vi "ZedBoardControlsTrippleSwitches.vi"(8 "Str Refnum":refnum<vi>, 9 "Bool Refnum":refnum<vi>, 10 "error out":errorcluster, 11 "queue out":refnum<queue>) -> ()   [LabVIEW 2012]
panel:
  in  "Sync Test\nMode Config":u32
  in  "Pulse Period\n(clock cycles -1)":u32
  in  "Channel \nMux Selector":bool
  in  "Channel \nHold Order":bool
  in  "Channel \nTransfer Order":bool
  in  "Throttle Mode":string(combo)
  in  "Sync Test Mode Select":string(combo)
  in  "Data Input Test Mode":string(combo)
  out "Last Command Sent":string
  out "state 34":bool
  out "state 33":bool
  out "state 32":bool
  in  "Sync2 3B":bool
  in  "Sync1 3B":bool
  in  "Sync0 3B":bool
  out "state 31":bool
  out "state 30":bool
  out "state 29":bool
  in  "Sync2 2B":bool
  in  "Sync1 2B":bool
  in  "Sync0 2B":bool
  out "state 28":bool
  out "state 27":bool
  out "state 26":bool
  in  "Sync2 1B":bool
  in  "Sync1 1B":bool
  in  "Sync0 1B":bool
  out "state 25":bool
  out "state 24":bool
  out "state 23":bool
  in  "Sync2 0B":bool
  in  "Sync1 0B":bool
  in  "Sync0 0B":bool
  out "state 22":bool
  out "state 21":bool
  out "state 20":bool
  in  "Sync2 7":bool
  in  "Sync1 7":bool
  in  "Sync0 7":bool
  out "state 19":bool
  out "state 18":bool
  out "state 17":bool
  in  "Sync2 6":bool
  in  "Sync1 6":bool
  in  "Sync0 6":bool
  out "state 16":bool
  out "state 15":bool
  out "state 14":bool
  in  "Sync2 5":bool
  in  "Sync1 5":bool
  in  "Sync0 5":bool
  out "state 13":bool
  out "state 12":bool
  out "state 11":bool
  in  "Sync2 4":bool
  in  "Sync1 4":bool
  in  "Sync0 4":bool
  out "state 10":bool
  out "state 9":bool
  out "state 8":bool
  in  "Sync2 3A":bool
  in  "Sync13A":bool
  in  "Sync0 3A":bool
  out "state 7":bool
  out "state 6":bool
  out "state 5":bool
  in  "Sync2 2A":bool
  in  "Sync1 2A":bool
  in  "Sync0 2A":bool
  out "state 4":bool
  out "state 2":bool
  out "state 3":bool
  in  "Sync2 1A":bool
  in  "Sync1 1A":bool
  in  "Sync0 1A":bool
  out "state":bool
  out "state 35":bool
  out "state 36":bool
  in  "Sync2 0A":bool
  in  "Sync1 0A":bool
  in  "Sync0 0A":bool
  in  "Reset Channel Enable":bool
  in  "Send Command, manual entry":string
  in  "Send":bool
  in  "Read Register":bool
  in  "Reset Register Map to Defaults":bool
  in  "Sync Enable":bool[](array[boolean])
  in  "Channel Enable":bool[](array[boolean])
  in  "Reset Profile Accumulator":bool[](array[boolean])
  in  "Counts Per Bin":u16
  in  "User Reset":bool
  in  "Number of Bins":u16
  in  "Profiles Per Histogram":u16
  in  "Time Reset":bool
  in  "Relative Time Step":u32
  in  "Demux Channel Enable":bool[](array[boolean])
  out "word0":string
  out "word1":string
  out "word2":string
  out "word3":string
  out "word4":string
  out "word5":string
  out "word6":string
  out "word7":string
  out "word8":string
  in  "Channel Polarization":bool[](array[boolean])
  in  "Demux Polarization":bool[](array[boolean])
  in  "Sync Polarization":bool[](array[boolean])
  in  "PIN0 Pulse Durration Ave 2^N":u16
  out "word9":string
  in  "PIN1 Pulse Durration Ave 2^N":u16
  in  "PIN2 Pulse Durration Ave 2^N":u16
  in  "PIN3 Pulse Durration Ave 2^N":u16
  in  "PIN4 Pulse Durration Ave 2^N":u16
  in  "PIN5 Pulse Durration Ave 2^N":u16
  in  "Send Word 0":bool
  in  "Send Word 1":bool
  in  "Send Word 2":bool
  in  "Send Word 3":bool
  in  "Send Word 4":bool
  in  "Send Word 5":bool
  in  "Send Word 6":bool
  in  "Send Word 7":bool
  in  "Send Word 8":bool
  in  "Send Word 9":bool
  # "word0"
  # "word1"
  # "word2"
  # "word3"
  # "word4"
  # "valid range (2-4096)"
  # "valid range (2-4096)"
  # "valid range (1-32,768)"
  # "word6"
  # "valid range (0-256)"
  # "valid range (0-128)"
  # "word7"
  # "word8"
  # "valid range (0-33,554,432)"
  # "word9"
  # "N=valid range (0-15)"
  # "N=valid range (0-15)"
  # "N=valid range (0-15)"
  # "N=valid range (0-15)"
  # "N=valid range (0-15)"
  # "N=valid range (0-15)"
  # "word5"
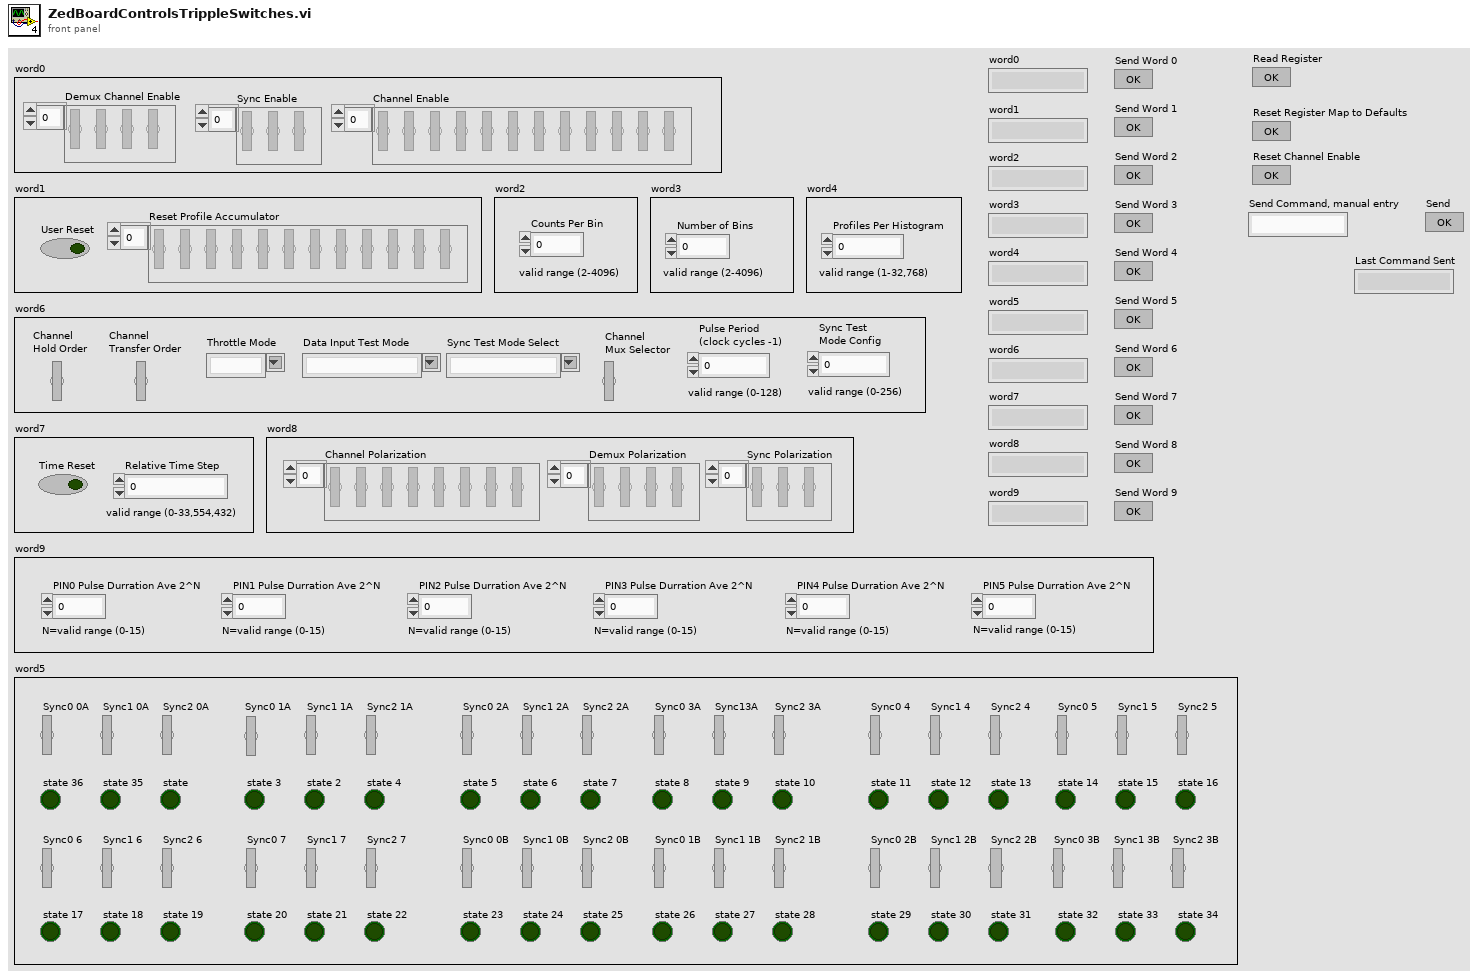
[diagram p1: front panel]
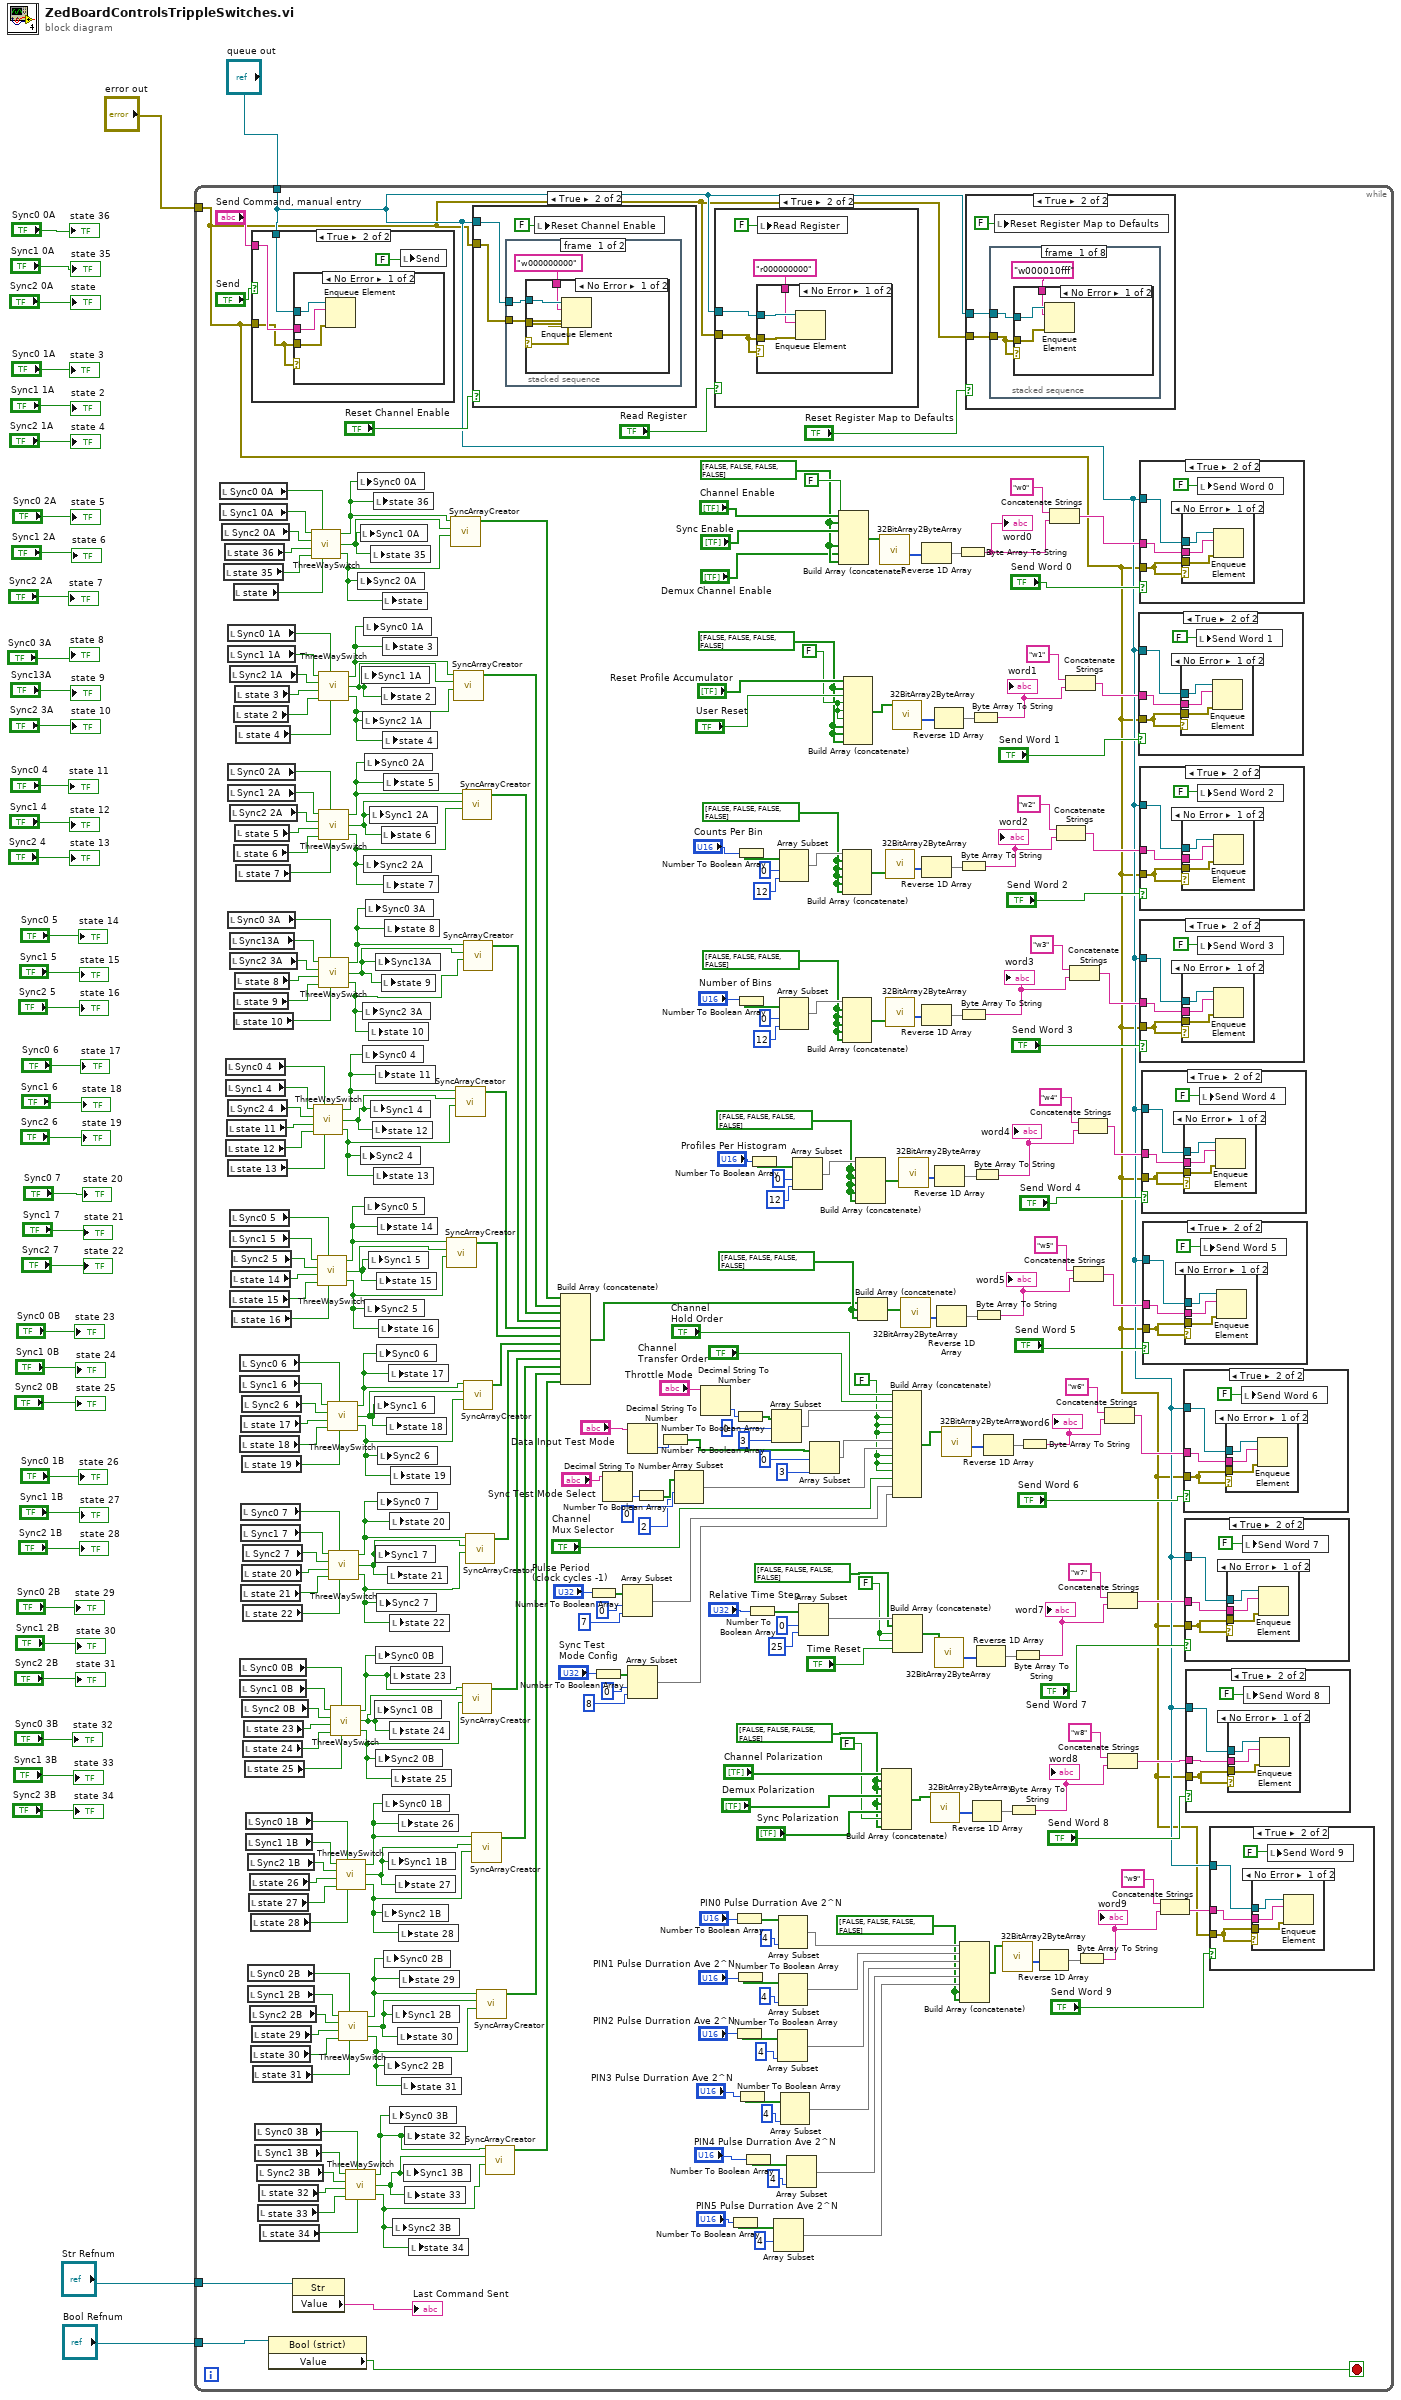
[diagram p0: block diagram]
diagram:
  n1 = while {
    tunnel: "queue out" -> [w200]
    tunnel: "error out" -> [w198]
    tunnel: "Bool Refnum" -> [w75]
    tunnel: "Str Refnum" -> [w73]
    stop <- w74 stop-if-true
    w239 = bool[] [FALSE, FALSE, FALSE, FALSE] ("appended array")
    w266 = bool[] [FALSE, FALSE, FALSE, FALSE] ("appended array")
    w275 = FALSE ("Read Register")
    w48 = FALSE ("Read Register")
    w287 = bool[] [FALSE, FALSE, FALSE, FALSE] ("appended array")
    w283 = bool[] [FALSE, FALSE, FALSE, FALSE] ("appended array")
    w284 = bool[] [FALSE, FALSE, FALSE, FALSE] ("appended array")
    w285 = bool[] [FALSE, FALSE, FALSE, FALSE] ("appended array")
    w311 = FALSE ("Read Register")
    w310 = bool[] [FALSE, FALSE, FALSE, FALSE] ("appended array")
    w320 = bool[] [FALSE, FALSE, FALSE, FALSE] ("appended array")
    n2 = local read "Sync0 0A"() -> (w170:bool)
    n3 = local read "Sync1 0A"() -> (w171:bool)
    n4 = local read "Sync2 0A"() -> (w172:bool)
    n5 = local read "state 35"() -> (w168:bool)
    n6 = local read "state 36"() -> (w167:bool)
    n7 = local read "Sync0 4"() -> (w175:bool)
    n8 = local read "Sync1 4"() -> (w174:bool)
    n9 = local read "state 12"() -> (w177:bool)
    n10 = local read "state 11"() -> (w178:bool)
    n11 = local read "Sync0 1A"() -> (w194:bool)
    n12 = local read "Sync1 1A"() -> (w195:bool)
    n13 = local read "Sync0 2A"() -> (w187:bool)
    n14 = local read "Sync1 2A"() -> (w186:bool)
    n15 = local read "Sync0 3A"() -> (w181:bool)
    n16 = local read "Sync2 4"() -> (w173:bool)
    n17 = local read "state 13"() -> (w176:bool)
    n18 = local read "Sync2 1A"() -> (w196:bool)
    n19 = local read "Sync2 2A"() -> (w185:bool)
    n20 = local read "Sync13A"() -> (w180:bool)
    n21 = local read "Sync2 3A"() -> (w179:bool)
    n22 = local read "Sync0 5"() -> (w164:bool)
    n23 = local read "Sync1 5"() -> (w165:bool)
    n24 = local read "state 15"() -> (w162:bool)
    n25 = local read "state 14"() -> (w161:bool)
    n26 = local read "Sync2 5"() -> (w166:bool)
    n27 = local read "state 16"() -> (w163:bool)
    n28 = local read "state"() -> (w169:bool)
    n29 = local read "state 10"() -> (w182:bool)
    n30 = local read "state 2"() -> (w192:bool)
    n31 = local read "state 6"() -> (w189:bool)
    n32 = local read "state 9"() -> (w183:bool)
    n33 = local read "state 3"() -> (w191:bool)
    n34 = local read "state 5"() -> (w190:bool)
    n35 = local read "state 8"() -> (w184:bool)
    n36 = local read "state 4"() -> (w193:bool)
    n37 = local read "state 7"() -> (w188:bool)
    n38 = local read "Sync0 6"() -> (w157:bool)
    n39 = local read "Sync1 6"() -> (w156:bool)
    n40 = local read "state 18"() -> (w159:bool)
    n41 = local read "Sync0 0B"() -> (w145:bool)
    n42 = local read "Sync1 0B"() -> (w144:bool)
    n43 = local read "state 17"() -> (w160:bool)
    n44 = local read "Sync0 7"() -> (w152:bool)
    n45 = local read "Sync1 7"() -> (w153:bool)
    n46 = local read "state 21"() -> (w150:bool)
    n47 = local read "Sync2 6"() -> (w155:bool)
    n48 = local read "state 19"() -> (w158:bool)
    n49 = local read "state 20"() -> (w149:bool)
    n50 = local read "Sync2 0B"() -> (w143:bool)
    n51 = local read "Sync2 7"() -> (w154:bool)
    n52 = local read "state 22"() -> (w151:bool)
    n53 = local read "state 24"() -> (w147:bool)
    n54 = local read "state 23"() -> (w148:bool)
    n55 = local read "state 25"() -> (w146:bool)
    n56 = local read "Sync0 1B"() -> (w140:bool)
    n57 = local read "Sync1 1B"() -> (w141:bool)
    n58 = local read "Sync2 1B"() -> (w142:bool)
    n59 = local read "Sync0 2B"() -> (w133:bool)
    n60 = local read "Sync1 2B"() -> (w132:bool)
    n61 = local read "state 27"() -> (w138:bool)
    n62 = local read "state 26"() -> (w137:bool)
    n63 = local read "Sync2 2B"() -> (w131:bool)
    n64 = local read "state 28"() -> (w139:bool)
    n65 = local read "state 30"() -> (w135:bool)
    n66 = case shown="True" "Send" {
      tunnel: "Send Command, manual entry" -> [_ w487]
      tunnel: w200 -> [_ w486]
      tunnel: w198 -> [_ w484]
      frame False {
      }
      frame True {
        n67 = case shown="No Error" w484 {
          tunnel: w487 -> [w490 _]
          tunnel: w484 -> [w489 _]
          tunnel: w486 -> [w488 _]
          frame No Error {
            n68 = Enqueue Element(queue=w488, element=w490, error in (no error)=w489) -> ()  [unwired: 1 in, 3 out]
          }
          frame Error {
          }
        }
        n69 = local write "Send"(FALSE ("Send")) -> ()
      }
    }
    n70 = local read "state 29"() -> (w136:bool)
    n71 = local read "state 31"() -> (w134:bool)
    n72 = local read "Sync0 3B"() -> (w128:bool)
    n73 = local read "Sync1 3B"() -> (w129:bool)
    n74 = local read "Sync2 3B"() -> (w130:bool)
    n75 = local read "state 33"() -> (w126:bool)
    n76 = local read "state 32"() -> (w125:bool)
    n77 = local read "state 34"() -> (w127:bool)
    n78 = property class="Bool (strict)"(reference=w75) -> ("Value"=w74:bool)  [unwired: 1 in, 2 out]
    n79 = property class="Str"(reference=w73) -> ("Value"=→"Last Command Sent":string)  [unwired: 1 in, 2 out]
    n80 = call "ThreeWaySwitch.vi"("Sync1"=w171, "Sync0"=w170, "Sync2"=w172, "Sync0 last state"=w167, "Sync2 last state"=w169, "Sync1 last state"=w168) -> ("Sync0out"=w124:bool, "Sync1out"=w123:bool, "Sync2out"=w122:bool)
    n81 = call "ThreeWaySwitch.vi"("Sync1"=w174, "Sync0"=w175, "Sync2"=w173, "Sync0 last state"=w178, "Sync2 last state"=w176, "Sync1 last state"=w177) -> ("Sync0out"=w112:bool, "Sync1out"=w111:bool, "Sync2out"=w110:bool)
    n82 = call "ThreeWaySwitch.vi"("Sync1"=w165, "Sync0"=w164, "Sync2"=w166, "Sync0 last state"=w161, "Sync2 last state"=w163, "Sync1 last state"=w162) -> ("Sync0out"=w109:bool, "Sync1out"=w108:bool, "Sync2out"=w107:bool)
    n83 = call "ThreeWaySwitch.vi"("Sync1"=w195, "Sync0"=w194, "Sync2"=w196, "Sync0 last state"=w191, "Sync2 last state"=w193, "Sync1 last state"=w192) -> ("Sync0out"=w119:bool, "Sync1out"=w120:bool, "Sync2out"=w121:bool)
    n84 = call "ThreeWaySwitch.vi"("Sync1"=w186, "Sync0"=w187, "Sync2"=w185, "Sync0 last state"=w190, "Sync2 last state"=w188, "Sync1 last state"=w189) -> ("Sync0out"=w118:bool, "Sync1out"=w117:bool, "Sync2out"=w116:bool)
    n85 = call "ThreeWaySwitch.vi"("Sync1"=w180, "Sync0"=w181, "Sync2"=w179, "Sync0 last state"=w184, "Sync2 last state"=w182, "Sync1 last state"=w183) -> ("Sync0out"=w115:bool, "Sync1out"=w114:bool, "Sync2out"=w113:bool)
    n86 = call "ThreeWaySwitch.vi"("Sync1"=w156, "Sync0"=w157, "Sync2"=w155, "Sync0 last state"=w160, "Sync2 last state"=w158, "Sync1 last state"=w159) -> ("Sync0out"=w106:bool, "Sync1out"=w105:bool, "Sync2out"=w104:bool)
    n87 = call "ThreeWaySwitch.vi"("Sync1"=w153, "Sync0"=w152, "Sync2"=w154, "Sync0 last state"=w149, "Sync2 last state"=w151, "Sync1 last state"=w150) -> ("Sync0out"=w103:bool, "Sync1out"=w102:bool, "Sync2out"=w101:bool)
    n88 = call "ThreeWaySwitch.vi"("Sync1"=w144, "Sync0"=w145, "Sync2"=w143, "Sync0 last state"=w148, "Sync2 last state"=w146, "Sync1 last state"=w147) -> ("Sync0out"=w100:bool, "Sync1out"=w99:bool, "Sync2out"=w98:bool)
    n89 = call "ThreeWaySwitch.vi"("Sync1"=w141, "Sync0"=w140, "Sync2"=w142, "Sync0 last state"=w137, "Sync2 last state"=w139, "Sync1 last state"=w138) -> ("Sync0out"=w97:bool, "Sync1out"=w96:bool, "Sync2out"=w95:bool)
    n90 = call "ThreeWaySwitch.vi"("Sync1"=w132, "Sync0"=w133, "Sync2"=w131, "Sync0 last state"=w136, "Sync2 last state"=w134, "Sync1 last state"=w135) -> ("Sync0out"=w94:bool, "Sync1out"=w93:bool, "Sync2out"=w92:bool)
    n91 = call "ThreeWaySwitch.vi"("Sync1"=w129, "Sync0"=w128, "Sync2"=w130, "Sync0 last state"=w125, "Sync2 last state"=w127, "Sync1 last state"=w126) -> ("Sync0out"=w91:bool, "Sync1out"=w90:bool, "Sync2out"=w89:bool)
    n92 = local write "Sync0 0A"(w124) -> ()
    n93 = local write "Sync2 0A"(w122) -> ()
    n94 = local write "Sync1 0A"(w123) -> ()
    n95 = local write "Sync2 4"(w110) -> ()
    n96 = local write "Sync1 1A"(w120) -> ()
    n97 = local write "Sync2 1A"(w121) -> ()
    n98 = local write "Sync2 3A"(w113) -> ()
    n99 = local write "Sync0 4"(w112) -> ()
    n100 = local write "Sync0 1A"(w119) -> ()
    n101 = local write "Sync2 2A"(w116) -> ()
    n102 = local write "Sync0 2A"(w118) -> ()
    n103 = local write "Sync0 5"(w109) -> ()
    n104 = local write "Sync2 5"(w107) -> ()
    n105 = local write "Sync0 3A"(w115) -> ()
    n106 = local write "state 10"(w113) -> ()
    n107 = local write "Sync1 5"(w108) -> ()
    n108 = local write "Sync1 2A"(w117) -> ()
    n109 = local write "state 35"(w123) -> ()
    n110 = local write "Sync1 4"(w111) -> ()
    n111 = local write "state 12"(w111) -> ()
    n112 = local write "state 36"(w124) -> ()
    n113 = local write "state 13"(w110) -> ()
    n114 = local write "Sync1 6"(w105) -> ()
    n115 = local write "Sync1 0B"(w99) -> ()
    n116 = local write "Sync13A"(w114) -> ()
    n117 = local write "state 11"(w112) -> ()
    n118 = local write "Sync1 7"(w102) -> ()
    n119 = local write "Sync0 0B"(w100) -> ()
    n120 = local write "Sync2 0B"(w98) -> ()
    n121 = local write "state 15"(w108) -> ()
    n122 = local write "Sync0 6"(w106) -> ()
    n123 = local write "Sync2 7"(w101) -> ()
    n124 = local write "state 14"(w109) -> ()
    n125 = local write "Sync2 6"(w104) -> ()
    n126 = local write "Sync0 7"(w103) -> ()
    n127 = local write "state 16"(w107) -> ()
    n128 = local write "state 2"(w120) -> ()
    n129 = local write "state 6"(w117) -> ()
    n130 = local write "state 9"(w114) -> ()
    n131 = local write "state"(w122) -> ()
    n132 = local write "Sync2 1B"(w95) -> ()
    n133 = local write "state 3"(w119) -> ()
    n134 = local write "state 4"(w121) -> ()
    n135 = local write "Sync0 1B"(w97) -> ()
    n136 = local write "state 5"(w118) -> ()
    n137 = local write "state 7"(w116) -> ()
    n138 = local write "Sync0 2B"(w94) -> ()
    n139 = local write "state 8"(w115) -> ()
    n140 = local write "Sync2 2B"(w92) -> ()
    n141 = local write "state 18"(w105) -> ()
    n142 = local write "state 21"(w102) -> ()
    n143 = local write "state 17"(w106) -> ()
    n144 = local write "Sync1 1B"(w96) -> ()
    n145 = local write "state 20"(w103) -> ()
    n146 = local write "state 22"(w101) -> ()
    n147 = local write "state 24"(w99) -> ()
    n148 = local write "Sync0 3B"(w91) -> ()
    n149 = local write "state 19"(w104) -> ()
    n150 = local write "state 23"(w100) -> ()
    n151 = local write "state 25"(w98) -> ()
    n152 = local write "Sync1 2B"(w93) -> ()
    n153 = local write "Sync2 3B"(w89) -> ()
    n154 = local write "state 27"(w96) -> ()
    n155 = local write "state 30"(w93) -> ()
    n156 = local write "state 26"(w97) -> ()
    n157 = local write "state 28"(w95) -> ()
    n158 = local write "state 29"(w94) -> ()
    n159 = local write "state 31"(w92) -> ()
    n160 = local write "Sync1 3B"(w90) -> ()
    n161 = local write "state 32"(w91) -> ()
    n162 = local write "state 33"(w90) -> ()
    n163 = local write "state 34"(w89) -> ()
    n164 = call "SyncArrayCreator.vi"("Sync2"=w107, "Sync1"=w108, "Sync0"=w109) -> ("Array"=w83:bool[])  [unwired: 8 in]
    n165 = call "SyncArrayCreator.vi"("Sync2"=w122, "Sync1"=w123, "Sync0"=w124) -> ("Array"=w88:bool[])  [unwired: 8 in]
    n166 = call "SyncArrayCreator.vi"("Sync2"=w121, "Sync1"=w120, "Sync0"=w119) -> ("Array"=w87:bool[])  [unwired: 8 in]
    n167 = call "SyncArrayCreator.vi"("Sync2"=w110, "Sync1"=w111, "Sync0"=w112) -> ("Array"=w84:bool[])  [unwired: 8 in]
    n168 = call "SyncArrayCreator.vi"("Sync2"=w116, "Sync1"=w117, "Sync0"=w118) -> ("Array"=w86:bool[])  [unwired: 8 in]
    n169 = call "SyncArrayCreator.vi"("Sync2"=w98, "Sync1"=w99, "Sync0"=w100) -> ("Array"=w80:bool[])  [unwired: 8 in]
    n170 = call "SyncArrayCreator.vi"("Sync2"=w113, "Sync1"=w114, "Sync0"=w115) -> ("Array"=w85:bool[])  [unwired: 8 in]
    n171 = call "SyncArrayCreator.vi"("Sync2"=w104, "Sync1"=w105, "Sync0"=w106) -> ("Array"=w82:bool[])  [unwired: 8 in]
    n172 = call "SyncArrayCreator.vi"("Sync2"=w101, "Sync1"=w102, "Sync0"=w103) -> ("Array"=w81:bool[])  [unwired: 8 in]
    n173 = call "SyncArrayCreator.vi"("Sync2"=w95, "Sync1"=w96, "Sync0"=w97) -> ("Array"=w79:bool[])  [unwired: 8 in]
    n174 = case shown="True" "Reset Channel Enable" {
      tunnel: w198 -> [_ w469]
      tunnel: w200 -> [_ w470]
      frame False {
      }
      frame True {
        n175 = stacked-sequence {
          tunnel: w469 -> [w474 w479]
          tunnel: w470 -> [w472 w478]
          frame #0 {
            n176 = case shown="No Error" w474 {
              tunnel: w474 -> [w477 _]
              tunnel: w472 -> [w476 _]
              tunnel: "w000000000" ("F-format string") -> [w475 _]
              frame No Error {
                n177 = Enqueue Element(queue=w476, element=w475, error in (no error)=w477) -> ()  [unwired: 1 in, 3 out]
              }
              frame Error {
              }
            }
          }
          frame #1 {
            n178 = case shown="No Error" w479 {
              tunnel: "w000010fff" ("F-format string") -> [w483 _]
              tunnel: w478 -> [w482 _]
              tunnel: w479 -> [w481 _]
              frame No Error {
                n179 = Enqueue Element(queue=w482, element=w483, error in (no error)=w481) -> ()  [unwired: 1 in, 3 out]
              }
              frame Error {
              }
            }
          }
        }
        n180 = local write "Reset Channel Enable"(FALSE ("Reset")) -> ()
      }
    }
    n181 = call "SyncArrayCreator.vi"("Sync2"=w92, "Sync1"=w93, "Sync0"=w94) -> ("Array"=w78:bool[])  [unwired: 8 in]
    n182 = call "SyncArrayCreator.vi"("Sync2"=w89, "Sync1"=w90, "Sync0"=w91) -> ("Array"=w77:bool[])  [unwired: 8 in]
    n183 = Build Array (concatenate)(w88, w87, w86, w85, w84, w83, w82, w81, w80, w79, w78, w77) -> (w76:bool[])
    n184 = Number To Boolean Array(number="Pulse Period\n(clock cycles -1)") -> (Boolean array=w59:bool[])
    n185 = Number To Boolean Array(number="Sync Test\nMode Config") -> (Boolean array=w46:bool[])
    n186 = Decimal String To Number(string="Sync Test Mode Select") -> (number=w66:i32)  [unwired: 2 in, 1 out]
    n187 = Array Subset(array=w59, index=0, length=7) -> (w51:bool[])
    n188 = Decimal String To Number(string="Data Input Test Mode") -> (number=w67:i32)  [unwired: 2 in, 1 out]
    n189 = Array Subset(array=w46, index=0, length=8) -> (w42:bool[])
    n190 = Number To Boolean Array(number=w66) -> (Boolean array=w60:bool[])
    n191 = Number To Boolean Array(number=w67) -> (Boolean array=w61:bool[])
    n192 = Array Subset(array=w60, index=0, length=2) -> (w49:bool[])
    n193 = Decimal String To Number(string="Throttle Mode") -> (number=w70:i32)  [unwired: 2 in, 1 out]
    n194 = case shown="True" "Read Register" {
      tunnel: w200 -> [_ w464]
      tunnel: w198 -> [_ w463]
      frame False {
      }
      frame True {
        n195 = case shown="No Error" w463 {
          tunnel: w464 -> [w468 _]
          tunnel: w463 -> [w467 _]
          tunnel: "r000000000" ("F-format string") -> [w466 _]
          frame No Error {
            n196 = Enqueue Element(queue=w468, element=w466, error in (no error)=w467) -> ()  [unwired: 1 in, 3 out]
          }
          frame Error {
          }
        }
        n197 = local write "Read Register"(FALSE ("Read Register")) -> ()
      }
    }
    n198 = Number To Boolean Array(number="PIN5 Pulse Durration Ave 2^N") -> (Boolean array=w255:bool[])
    n199 = Number To Boolean Array(number="PIN0 Pulse Durration Ave 2^N") -> (Boolean array=w264:bool[])
    n200 = Number To Boolean Array(number="PIN2 Pulse Durration Ave 2^N") -> (Boolean array=w251:bool[])
    n201 = Number To Boolean Array(number=w70) -> (Boolean array=w330:bool[])
    n202 = Number To Boolean Array(number="PIN1 Pulse Durration Ave 2^N") -> (Boolean array=w259:bool[])
    n203 = Number To Boolean Array(number="Counts Per Bin") -> (Boolean array=w333:bool[])
    n204 = Number To Boolean Array(number="Number of Bins") -> (Boolean array=w304:bool[])
    n205 = Number To Boolean Array(number="PIN3 Pulse Durration Ave 2^N") -> (Boolean array=w253:bool[])
    n206 = Number To Boolean Array(number="PIN4 Pulse Durration Ave 2^N") -> (Boolean array=w257:bool[])
    n207 = Number To Boolean Array(number="Relative Time Step") -> (Boolean array=w327:bool[])
    n208 = Number To Boolean Array(number="Profiles Per Histogram") -> (Boolean array=w296:bool[])
    n209 = Array Subset(array=w330, index=0, length=3) -> (w55:bool[])
    n210 = Array Subset(array=w255, length=4) -> (w240:bool[])  [unwired: 1 in]
    n211 = Array Subset(array=w251, length=4) -> (w243:bool[])  [unwired: 1 in]
    n212 = Array Subset(array=w264, length=4) -> (w245:bool[])  [unwired: 1 in]
    n213 = Array Subset(array=w259, length=4) -> (w244:bool[])  [unwired: 1 in]
    n214 = Array Subset(array=w333, index=0, length=12) -> (w307:bool[])
    n215 = Array Subset(array=w304, index=0, length=12) -> (w300:bool[])
    n216 = Array Subset(array=w253, length=4) -> (w242:bool[])  [unwired: 1 in]
    n217 = Array Subset(array=w257, length=4) -> (w241:bool[])  [unwired: 1 in]
    n218 = Array Subset(array=w296, index=0, length=12) -> (w292:bool[])
    n219 = Array Subset(array=w327, index=0, length=25) -> (w277:bool[])
    n220 = Array Subset(array=w61, index=0, length=3) -> (w52:bool[])
    n221 = Build Array (concatenate)("Channel Enable", w320, "Sync Enable", FALSE ("Read Register"), w320, "Demux Channel Enable", w320) -> (w324:bool[])
    n222 = Build Array (concatenate)(w307, w285, w285, w285, w285, w285) -> (w286:bool[])
    n223 = Build Array (concatenate)(w300, w284, w284, w284, w284, w284) -> (w303:bool[])
    n224 = Build Array (concatenate)("Reset Profile Accumulator", w310, "User Reset", w311, w311, w311, w310, w310, w310) -> (w316:bool[])
    n225 = Build Array (concatenate)(w292, w283, w283, w283, w283, w283) -> (w295:bool[])
    n226 = Build Array (concatenate)(w76, w287, w287) -> (w290:bool[])
    n227 = call "32BitArray2ByteArray.vi"("Array in"=w324) -> ("Byte array out"=w318:u32[])  [unwired: 10 in]
    n228 = Build Array (concatenate)("Channel Polarization", w266, w266, "Demux Polarization", w266, "Sync Polarization", FALSE ("Read Register"), w266) -> (w273:bool[])
    n229 = call "32BitArray2ByteArray.vi"("Array in"=w286) -> ("Byte array out"=w309:u32[])  [unwired: 10 in]
    n230 = call "32BitArray2ByteArray.vi"("Array in"=w303) -> ("Byte array out"=w302:u32[])  [unwired: 10 in]
    n231 = call "32BitArray2ByteArray.vi"("Array in"=w316) -> ("Byte array out"=w315:u32[])  [unwired: 10 in]
    n232 = Build Array (concatenate)("Channel \nHold Order", "Channel \nTransfer Order", w55, w48, w48, w48, w52, w49, w48, w48, w48, "Channel \nMux Selector", w51, w42) -> (w47:bool[])
    n233 = Build Array (concatenate)(w277, bool[] [FALSE, FALSE, FALSE, FALSE] ("appended array"), w275, w275, "Time Reset") -> (w280:bool[])
    n234 = call "32BitArray2ByteArray.vi"("Array in"=w295) -> ("Byte array out"=w294:u32[])  [unwired: 10 in]
    n235 = call "32BitArray2ByteArray.vi"("Array in"=w290) -> ("Byte array out"=w289:u32[])  [unwired: 10 in]
    n236 = Reverse 1D Array(array=w318) -> (reversed array=w317:u32[])
    n237 = Reverse 1D Array(array=w309) -> (reversed array=w308:u32[])
    n238 = Reverse 1D Array(array=w302) -> (reversed array=w301:u32[])
    n239 = call "32BitArray2ByteArray.vi"("Array in"=w273) -> ("Byte array out"=w272:u32[])  [unwired: 10 in]
    n240 = Reverse 1D Array(array=w315) -> (reversed array=w314:u32[])
    n241 = call "32BitArray2ByteArray.vi"("Array in"=w280) -> ("Byte array out"=w279:u32[])  [unwired: 10 in]
    n242 = Reverse 1D Array(array=w294) -> (reversed array=w293:u32[])
    n243 = Reverse 1D Array(array=w289) -> (reversed array=w288:u32[])
    n244 = call "32BitArray2ByteArray.vi"("Array in"=w47) -> ("Byte array out"=w282:u32[])  [unwired: 10 in]
    n245 = Byte Array To String(unsigned byte array=w317) -> (string=w237:string)
    "word0" <- w237
    n246 = Byte Array To String(unsigned byte array=w308) -> (string=w222:string)
    "word2" <- w222
    n247 = Byte Array To String(unsigned byte array=w301) -> (string=w215:string)
    "word3" <- w215
    n248 = Build Array (concatenate)(w245, w244, w243, w242, w241, w240, w239, w239) -> (w263:bool[])
    n249 = case shown="True" "Reset Register Map to Defaults" {
      tunnel: w200 -> [_ w412]
      tunnel: w198 -> [_ w411]
      frame False {
      }
      frame True {
        n250 = stacked-sequence {
          tunnel: w412 -> [w416 w422 w428 w434 w440 w446 w452 w458]
          tunnel: w411 -> [w415 w421 w427 w433 w439 w445 w451 w457]
          frame #0 {
            n251 = case shown="No Error" w415 {
              tunnel: w416 -> [w419 _]
              tunnel: w415 -> [w418 _]
              tunnel: "w000010fff" ("F-format string") -> [w417 _]
              frame No Error {
                n252 = Enqueue Element(queue=w419, element=w417, error in (no error)=w418) -> ()  [unwired: 1 in, 3 out]
              }
              frame Error {
              }
            }
          }
          frame #1 {
            n253 = case shown="No Error" w421 {
              tunnel: w422 -> [w425 _]
              tunnel: w421 -> [w424 _]
              tunnel: "w100000000" ("F-format string") -> [w423 _]
              frame No Error {
                n254 = Enqueue Element(queue=w425, element=w423, error in (no error)=w424) -> ()  [unwired: 1 in, 3 out]
              }
              frame Error {
              }
            }
          }
          frame #2 {
            n255 = case shown="No Error" w427 {
              tunnel: w428 -> [w431 _]
              tunnel: w427 -> [w430 _]
              tunnel: "w20000000a" ("F-format string") -> [w429 _]
              frame No Error {
                n256 = Enqueue Element(queue=w431, element=w429, error in (no error)=w430) -> ()  [unwired: 1 in, 3 out]
              }
              frame Error {
              }
            }
          }
          frame #3 {
            n257 = case shown="No Error" w433 {
              tunnel: w434 -> [w437 _]
              tunnel: w433 -> [w436 _]
              tunnel: "w300000bb8" ("F-format string") -> [w435 _]
              frame No Error {
                n258 = Enqueue Element(queue=w437, element=w435, error in (no error)=w436) -> ()  [unwired: 1 in, 3 out]
              }
              frame Error {
              }
            }
          }
          frame #4 {
            n259 = case shown="No Error" w439 {
              tunnel: w440 -> [w443 _]
              tunnel: w439 -> [w442 _]
              tunnel: "w400002000" ("F-format string") -> [w441 _]
              frame No Error {
                n260 = Enqueue Element(queue=w443, element=w441, error in (no error)=w442) -> ()  [unwired: 1 in, 3 out]
              }
              frame Error {
              }
            }
          }
          frame #5 {
            n261 = case shown="No Error" w445 {
              tunnel: w446 -> [w449 _]
              tunnel: w445 -> [w448 _]
              tunnel: "w500000000" ("F-format string") -> [w447 _]
              frame No Error {
                n262 = Enqueue Element(queue=w449, element=w447, error in (no error)=w448) -> ()  [unwired: 1 in, 3 out]
              }
              frame Error {
              }
            }
          }
          frame #6 {
            n263 = case shown="No Error" w451 {
              tunnel: w452 -> [w455 _]
              tunnel: w451 -> [w454 _]
              tunnel: "w61f000a00" ("F-format string") -> [w453 _]
              frame No Error {
                n264 = Enqueue Element(queue=w455, element=w453, error in (no error)=w454) -> ()  [unwired: 1 in, 3 out]
              }
              frame Error {
              }
            }
          }
          frame #7 {
            n265 = case shown="No Error" w457 {
              tunnel: w458 -> [w461 _]
              tunnel: w457 -> [w460 _]
              tunnel: "w701312d00" ("F-format string") -> [w459 _]
              frame No Error {
                n266 = Enqueue Element(queue=w461, element=w459, error in (no error)=w460) -> ()  [unwired: 1 in, 3 out]
              }
              frame Error {
              }
            }
          }
        }
        n267 = local write "Reset Register Map to Defaults"(FALSE ("Read Register")) -> ()
      }
    }
    n268 = Byte Array To String(unsigned byte array=w314) -> (string=w225:string)
    "word1" <- w225
    n269 = Byte Array To String(unsigned byte array=w293) -> (string=w216:string)
    "word4" <- w216
    n270 = Reverse 1D Array(array=w272) -> (reversed array=w271:u32[])
    n271 = Byte Array To String(unsigned byte array=w288) -> (string=w217:string)
    "word5" <- w217
    n272 = Reverse 1D Array(array=w279) -> (reversed array=w278:u32[])
    n273 = Reverse 1D Array(array=w282) -> (reversed array=w281:u32[])
    n274 = call "32BitArray2ByteArray.vi"("Array in"=w263) -> ("Byte array out"=w262:u32[])  [unwired: 10 in]
    n275 = Byte Array To String(unsigned byte array=w271) -> (string=w220:string)
    "word8" <- w220
    n276 = Byte Array To String(unsigned byte array=w278) -> (string=w219:string)
    "word7" <- w219
    n277 = Byte Array To String(unsigned byte array=w281) -> (string=w218:string)
    "word6" <- w218
    n278 = Reverse 1D Array(array=w262) -> (reversed array=w261:u32[])
    n279 = Concatenate Strings("w0" ("string"), w237) -> (w236:string)
    n280 = Concatenate Strings("w2" ("string"), w222) -> (w214:string)
    n281 = Concatenate Strings("w1" ("string"), w225) -> (w223:string)
    n282 = Concatenate Strings("w3" ("string"), w215) -> (w213:string)
    n283 = Concatenate Strings("w5" ("string"), w217) -> (w211:string)
    n284 = Byte Array To String(unsigned byte array=w261) -> (string=w221:string)
    "word9" <- w221
    n285 = Concatenate Strings("w4" ("string"), w216) -> (w212:string)
    n286 = Concatenate Strings("w6" ("string"), w218) -> (w210:string)
    n287 = Concatenate Strings("w7" ("string"), w219) -> (w203:string)
    n288 = Concatenate Strings("w8" ("string"), w220) -> (w201:string)
    n289 = case shown="True" "Send Word 1" {
      tunnel: w223 -> [_ w400]
      tunnel: w200 -> [_ w399]
      tunnel: w198 -> [_ w397]
      frame False {
      }
      frame True {
        n290 = case shown="No Error" w397 {
          tunnel: w400 -> [w403 _]
          tunnel: w397 -> [w402 _]
          tunnel: w399 -> [w401 _]
          frame No Error {
            n291 = Enqueue Element(queue=w401, element=w403, error in (no error)=w402) -> ()  [unwired: 1 in, 3 out]
          }
          frame Error {
          }
        }
        n292 = local write "Send Word 1"(FALSE ("Send")) -> ()
      }
    }
    n293 = case shown="True" "Send Word 0" {
      tunnel: w236 -> [_ w407]
      tunnel: w200 -> [_ w406]
      tunnel: w198 -> [_ w404]
      frame False {
      }
      frame True {
        n294 = case shown="No Error" w404 {
          tunnel: w407 -> [w410 _]
          tunnel: w404 -> [w409 _]
          tunnel: w406 -> [w408 _]
          frame No Error {
            n295 = Enqueue Element(queue=w408, element=w410, error in (no error)=w409) -> ()  [unwired: 1 in, 3 out]
          }
          frame Error {
          }
        }
        n296 = local write "Send Word 0"(FALSE ("Send")) -> ()
      }
    }
    n297 = case shown="True" "Send Word 2" {
      tunnel: w214 -> [_ w393]
      tunnel: w200 -> [_ w392]
      tunnel: w198 -> [_ w390]
      frame False {
      }
      frame True {
        n298 = case shown="No Error" w390 {
          tunnel: w393 -> [w396 _]
          tunnel: w390 -> [w395 _]
          tunnel: w392 -> [w394 _]
          frame No Error {
            n299 = Enqueue Element(queue=w394, element=w396, error in (no error)=w395) -> ()  [unwired: 1 in, 3 out]
          }
          frame Error {
          }
        }
        n300 = local write "Send Word 2"(FALSE ("Send")) -> ()
      }
    }
    n301 = case shown="True" "Send Word 3" {
      tunnel: w213 -> [_ w386]
      tunnel: w200 -> [_ w385]
      tunnel: w198 -> [_ w383]
      frame False {
      }
      frame True {
        n302 = case shown="No Error" w383 {
          tunnel: w386 -> [w389 _]
          tunnel: w383 -> [w388 _]
          tunnel: w385 -> [w387 _]
          frame No Error {
            n303 = Enqueue Element(queue=w387, element=w389, error in (no error)=w388) -> ()  [unwired: 1 in, 3 out]
          }
          frame Error {
          }
        }
        n304 = local write "Send Word 3"(FALSE ("Send")) -> ()
      }
    }
    n305 = case shown="True" "Send Word 4" {
      tunnel: w212 -> [_ w379]
      tunnel: w200 -> [_ w378]
      tunnel: w198 -> [_ w376]
      frame False {
      }
      frame True {
        n306 = case shown="No Error" w376 {
          tunnel: w379 -> [w382 _]
          tunnel: w376 -> [w381 _]
          tunnel: w378 -> [w380 _]
          frame No Error {
            n307 = Enqueue Element(queue=w380, element=w382, error in (no error)=w381) -> ()  [unwired: 1 in, 3 out]
          }
          frame Error {
          }
        }
        n308 = local write "Send Word 4"(FALSE ("Send")) -> ()
      }
    }
    n309 = case shown="True" "Send Word 5" {
      tunnel: w211 -> [_ w372]
      tunnel: w200 -> [_ w371]
      tunnel: w198 -> [_ w369]
      frame False {
      }
      frame True {
        n310 = case shown="No Error" w369 {
          tunnel: w372 -> [w375 _]
          tunnel: w369 -> [w374 _]
          tunnel: w371 -> [w373 _]
          frame No Error {
            n311 = Enqueue Element(queue=w373, element=w375, error in (no error)=w374) -> ()  [unwired: 1 in, 3 out]
          }
          frame Error {
          }
        }
        n312 = local write "Send Word 5"(FALSE ("Send")) -> ()
      }
    }
    n313 = Concatenate Strings("w9" ("string"), w221) -> (w199:string)
    n314 = case shown="True" "Send Word 6" {
      tunnel: w210 -> [_ w365]
      tunnel: w200 -> [_ w364]
      tunnel: w198 -> [_ w362]
      frame False {
      }
      frame True {
        n315 = case shown="No Error" w362 {
          tunnel: w365 -> [w368 _]
          tunnel: w362 -> [w367 _]
          tunnel: w364 -> [w366 _]
          frame No Error {
            n316 = Enqueue Element(queue=w366, element=w368, error in (no error)=w367) -> ()  [unwired: 1 in, 3 out]
          }
          frame Error {
          }
        }
        n317 = local write "Send Word 6"(FALSE ("Send")) -> ()
      }
    }
    n318 = case shown="True" "Send Word 7" {
      tunnel: w203 -> [_ w358]
      tunnel: w200 -> [_ w357]
      tunnel: w198 -> [_ w355]
      frame False {
      }
      frame True {
        n319 = case shown="No Error" w355 {
          tunnel: w358 -> [w361 _]
          tunnel: w355 -> [w360 _]
          tunnel: w357 -> [w359 _]
          frame No Error {
            n320 = Enqueue Element(queue=w359, element=w361, error in (no error)=w360) -> ()  [unwired: 1 in, 3 out]
          }
          frame Error {
          }
        }
        n321 = local write "Send Word 7"(FALSE ("Send")) -> ()
      }
    }
    n322 = case shown="True" "Send Word 8" {
      tunnel: w201 -> [_ w351]
      tunnel: w200 -> [_ w350]
      tunnel: w198 -> [_ w348]
      frame False {
      }
      frame True {
        n323 = case shown="No Error" w348 {
          tunnel: w351 -> [w354 _]
          tunnel: w348 -> [w353 _]
          tunnel: w350 -> [w352 _]
          frame No Error {
            n324 = Enqueue Element(queue=w352, element=w354, error in (no error)=w353) -> ()  [unwired: 1 in, 3 out]
          }
          frame Error {
          }
        }
        n325 = local write "Send Word 8"(FALSE ("Send")) -> ()
      }
    }
    n326 = case shown="True" "Send Word 9" {
      tunnel: w199 -> [_ w344]
      tunnel: w200 -> [_ w343]
      tunnel: w198 -> [_ w341]
      frame False {
      }
      frame True {
        n327 = case shown="No Error" w341 {
          tunnel: w344 -> [w347 _]
          tunnel: w341 -> [w346 _]
          tunnel: w343 -> [w345 _]
          frame No Error {
            n328 = Enqueue Element(queue=w345, element=w347, error in (no error)=w346) -> ()  [unwired: 1 in, 3 out]
          }
          frame Error {
          }
        }
        n329 = local write "Send Word 9"(FALSE ("Send")) -> ()
      }
    }
  }
  "state 36" <- "Sync0 0A"
  "state 35" <- "Sync1 0A"
  "state" <- "Sync2 0A"
  "state 3" <- "Sync0 1A"
  "state 2" <- "Sync1 1A"
  "state 4" <- "Sync2 1A"
  "state 5" <- "Sync0 2A"
  "state 6" <- "Sync1 2A"
  "state 7" <- "Sync2 2A"
  "state 8" <- "Sync0 3A"
  "state 9" <- "Sync13A"
  "state 10" <- "Sync2 3A"
  "state 11" <- "Sync0 4"
  "state 12" <- "Sync1 4"
  "state 13" <- "Sync2 4"
  "state 14" <- "Sync0 5"
  "state 15" <- "Sync1 5"
  "state 16" <- "Sync2 5"
  "state 17" <- "Sync0 6"
  "state 18" <- "Sync1 6"
  "state 19" <- "Sync2 6"
  "state 20" <- "Sync0 7"
  "state 21" <- "Sync1 7"
  "state 22" <- "Sync2 7"
  "state 23" <- "Sync0 0B"
  "state 24" <- "Sync1 0B"
  "state 25" <- "Sync2 0B"
  "state 26" <- "Sync0 1B"
  "state 27" <- "Sync1 1B"
  "state 28" <- "Sync2 1B"
  "state 29" <- "Sync0 2B"
  "state 30" <- "Sync1 2B"
  "state 31" <- "Sync2 2B"
  "state 32" <- "Sync0 3B"
  "state 33" <- "Sync1 3B"
  "state 34" <- "Sync2 3B"
